vi "Voltage Output Test.vi"(8 "Error In":errorcluster, 9 "Line In":dbl, 10 "Power Supply In":string, 11 "DMM In":string) -> (0 "Error Out":errorcluster, 3 "Output Voltage":dbl)   [LabVIEW 2015]
doc: "Measures the output DC voltage when providing an input voltage from the battery pins."
uses:
  <instrlib>/Driver Simulation/DMM/Signal Types.ctl
  <instrlib>/Driver Simulation/Power Supply.lvlib
  <instrlib>/Driver Simulation/DMM.lvlib
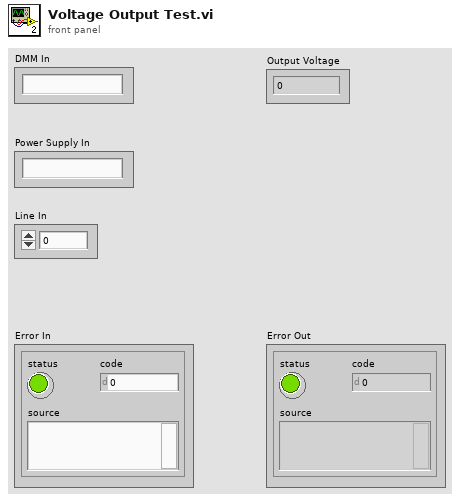
[diagram p1: front panel]
types:
  T1 = typedef "Driver Simulation.lvlib/DMM.lvlib/Signal Types.ctl" = enum16{"DC", "AC"}
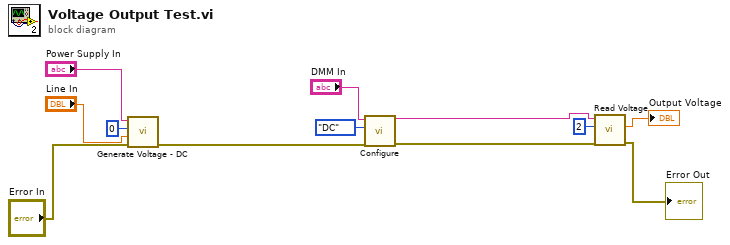
[diagram p0: block diagram]
diagram:
  n1 = call <instrlib>:"Generate Voltage - DC.vi"("error in (no error)"="Error In", "Output Voltage"="Line In", "Channel"=0, "Power Supply in"="Power Supply In") -> ("error out"=w10:errorcluster)  [unwired: 6 in, 1 out]
  n2 = call <instrlib>:"Configure.vi"("error in (no error)"=w10, "Signal Type"=Signal_Types."DC", "DMM in"="DMM In") -> ("error out"=w9:errorcluster, "DMM out"=w4:string)  [unwired: 7 in]
  n3 = call <instrlib>:"Read Voltage.vi"("error in (no error)"=w9, "Channel"=2, "DMM in"=w4) -> ("error out"=→"Error Out":errorcluster, "Voltage"=→"Output Voltage":dbl)  [unwired: 6 in, 1 out]
